vi "GOOP_DependencyViewer_ReadConfigFile.vi"() -> (3 "Config":T1)   [LabVIEW 2020]
uses:
  <resource>/Framework/Providers/Open_GDS/SubVIs/GOOP_DependencySettings.ctl
  <resource>/Framework/Providers/Open_GDS/DependencyViewer/DependencyChecker/DependencyConfiguration.ctl
  <resource>/Framework/Providers/Open_GDS/DependencyViewer/DependencyChecker/FilterOptions.ctl
  <resource>/Framework/Providers/Open_GDS/DependencyViewer/DependencyChecker/DependencyChecker.lvlib
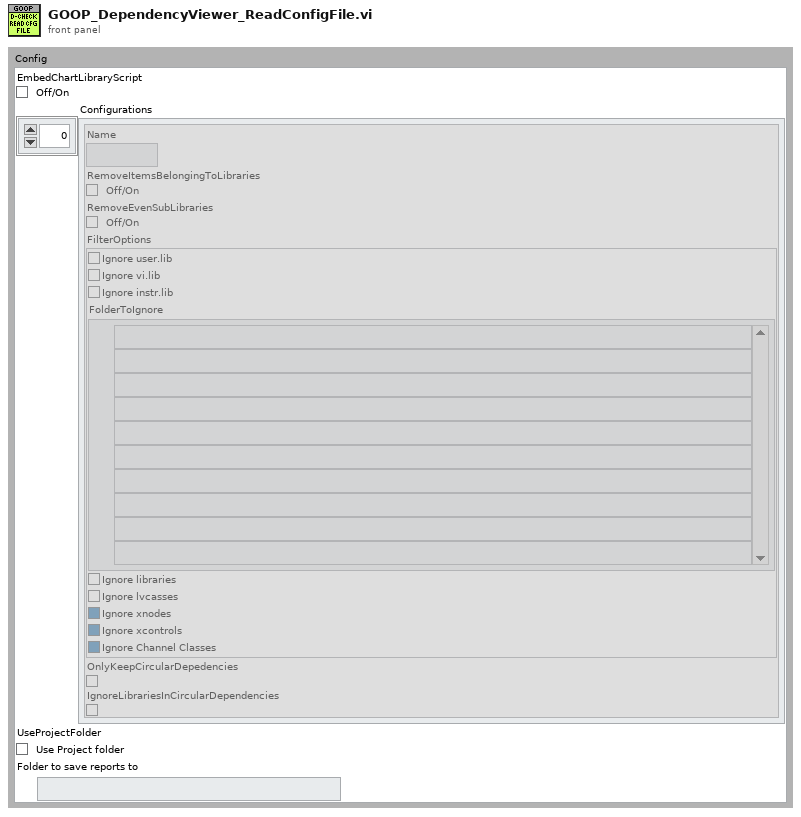
[diagram p1: front panel]
types:
  T1 = typedef "GOOP_DependencySettings.ctl" = cluster{"EmbedChartLibraryScript":bool, "Configurations":T2[], "UseProjectFolder":bool, "Folder to save reports to":path}
  T2 = typedef "DependencyChecker.lvlib/DependencyConfiguration.ctl" = cluster{"Name":string, "RemoveItemsBelongingToLibraries":bool, "RemoveEvenSubLibraries":bool, "FilterOptions":T3, "OnlyKeepCircularDepedencies":bool, "IgnoreLibrariesInCircularDependencies":bool}
  T3 = typedef "DependencyChecker.lvlib/FilterOptions.ctl" = cluster{"Ignore user.lib":bool, "Ignore vi.lib":bool, "Ignore instr.lib":bool, "FolderToIgnore":path[], "Ignore libraries":bool, "Ignore lvcasses":bool, "Ignore xnodes":bool, "Ignore xcontrols":bool, "Ignore Channel Classes":bool}
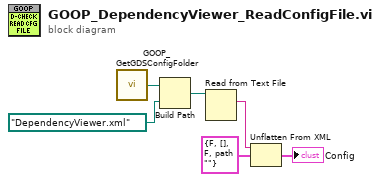
[diagram p0: block diagram]
diagram:
  n1 = call <resource>:"GOOP_GetGDSConfigFolder.vi"() -> ("GDSFolderPath"=w5:path)
  n2 = Build Path(base path=w5, name or relative path=path "DependencyViewer.xml") -> (appended path=w4:path)
  n3 = Read from Text File(file (use dialog)=w4) -> (text=w6:string)  [unwired: 3 in, 3 out]
  n4 = Unflatten From XML(xml string=w6, type=T1 {"EmbedChartLibraryScript"=FALSE, "Configurations"=[], "UseProjectFolder"=FALSE, "Folder to save reports to"=path ""}) -> (value=→"Config":T1)  [unwired: 1 in, 1 out]
